vi "Read Namer.vi"(8 "error in":errorcluster, 11 "Options in":refnum<class "Options.lvclass">) -> (0 "error out":errorcluster, 2 "Approval Tests.lvlib:Namer.lvclass":refnum<class "Namer.lvclass">, 3 "Options out":refnum<class "Options.lvclass">)   [LabVIEW 2020, in "Approval Tests.lvlib" / "Options.lvclass"]
uses:
  Options.lvclass
  Namer/Namer.lvclass
  Options.lvclass/Options.ctl
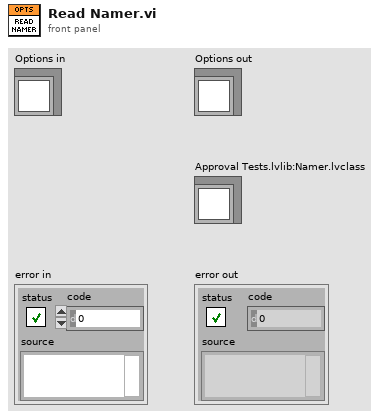
[diagram p1: front panel]
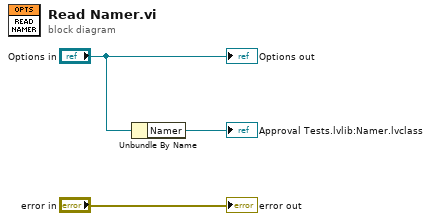
[diagram p0: block diagram]
diagram:
  n1 = Unbundle By Name("Options in") -> ("Namer"=→"Approval Tests.lvlib:Namer.lvclass":refnum<class "Namer.lvclass">)
  "error out" <- "error in"
  "Options out" <- "Options in"
